vi "Main.vi"() -> ()   [LabVIEW 2017]
doc: "This Continuous Measurement sample project is based on the Queued Message Handler template.\n\nThe Event Handling Loop generates messages based on user interface actions.\n\nThe Message Handling Loop processes messages generated by the Event Handling Loop, or by other messages. There are also Acquisition and Logging message handling loop subVIs, and a chart updating loop."
uses:
  Settings/Settings.ctl
  Acquisition/Hardware Configuration.ctl
  Acquisition/Signal Type.ctl
  Logging/Logging Configuration.ctl
  controls/UI Data.ctl
  controls/UI State.ctl
  3e1da0e8-c032-3fe2-cb30-6c3ce3a1e83f.vi
  support/Message Queue/Enqueue Message (Single).vi
  support/Message Queue/Enqueue Message (Array).vi
  <vilib>/Utility/error.llb/Error Cluster From Error Code.vi
  <vilib>/ErrorRing/Error Ring.xnode
  Acquisition/Acquisition.lvlib
  Logging/Logging.lvlib
  Settings/Settings.lvlib
  support/User Event - Stop/User Event - Stop.lvlib
  support/Message Queue/Message Queue.lvlib
  Settings/Settings Dialog.vi
panel:
  out "Zero run":bool
  in  "Zero run?":bool
  out "Max writing time to a file [min]":dbl
  out "Elapsed time":timestamp
  out "Test time zero run [s]":dbl
  out "Test time [s]":dbl
  in  "Start":bool
  in  "Stop":bool
  in  "Settings":bool
  out "Status":string
  in  "Exit":bool
  out "Log File Offsite Path":path
  out "Project code":string
  out "Offsite storage?":bool
  out "Log File Path":path
  out "Data":waveform(dbl)[](graph)
  # "Continuous Measurement Data Logger"
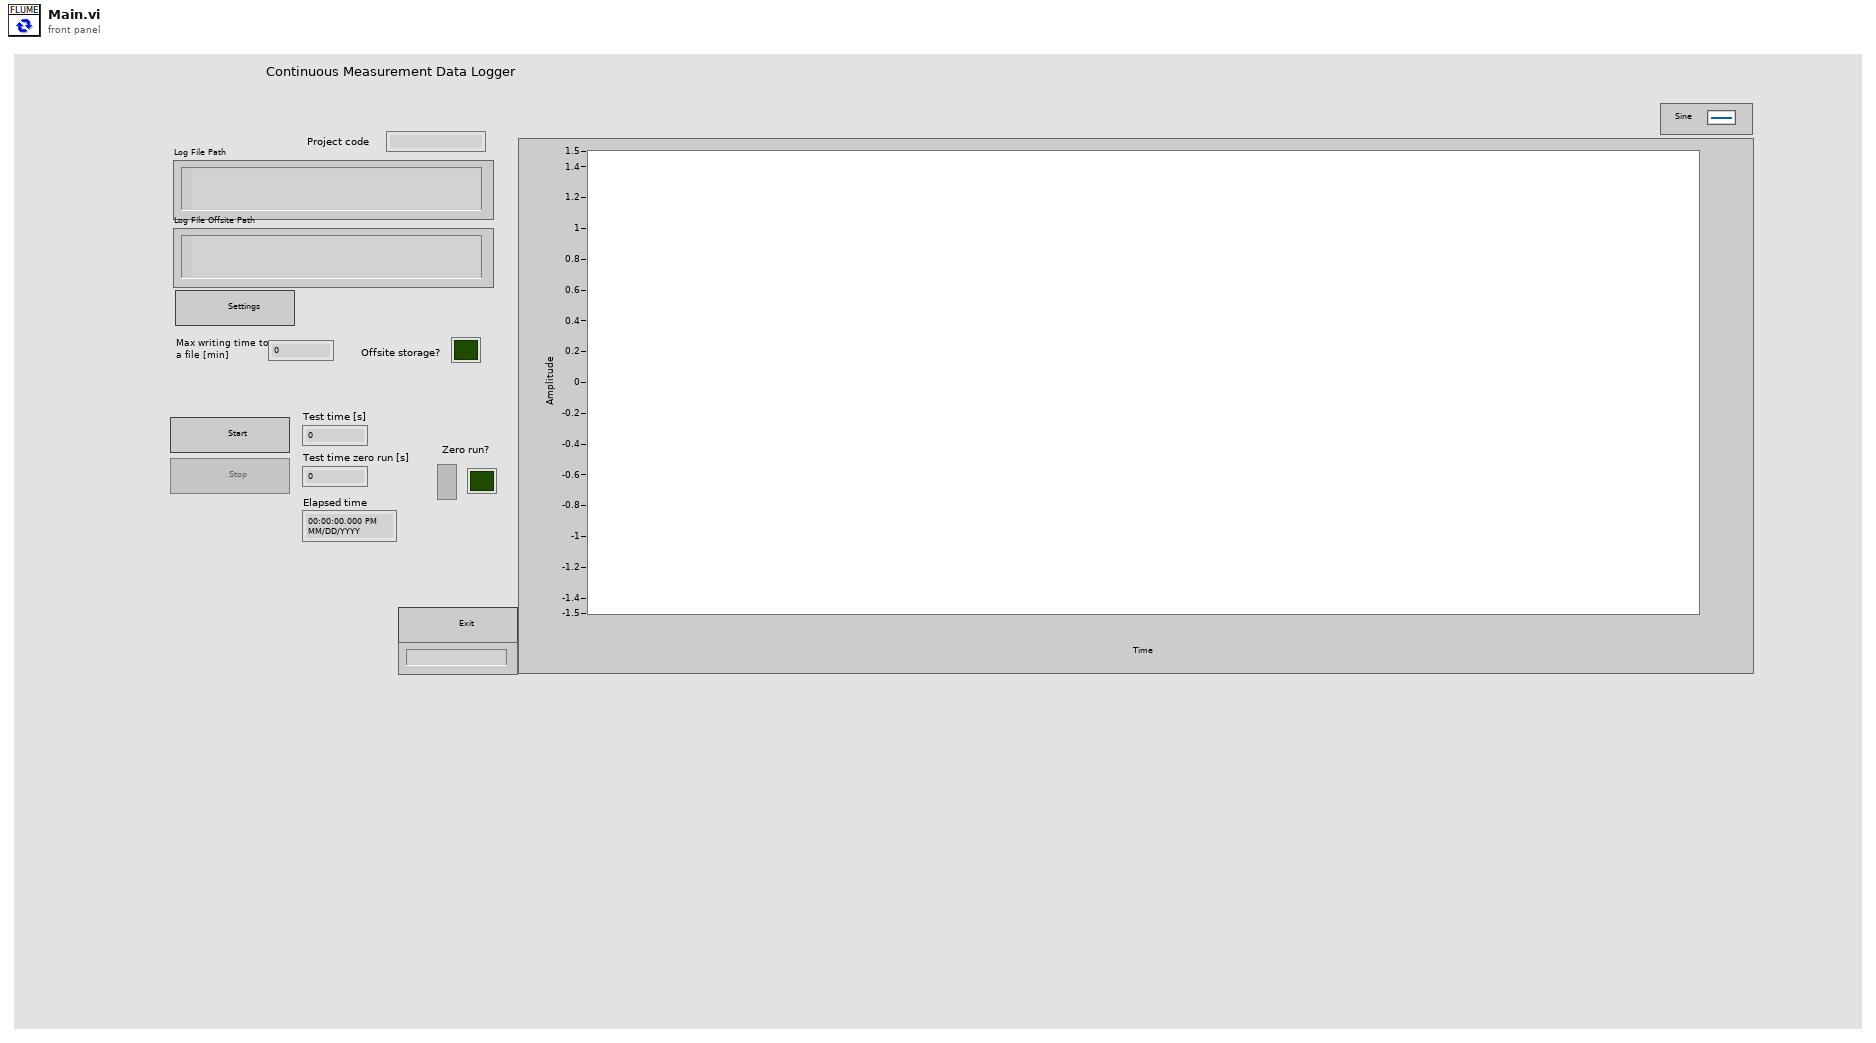
[diagram p1: front panel]
types:
  T1 = typedef "UI State.ctl" = enum16{"Idle", "Acquiring and Logging", "Waiting for Exit", "Waiting for Exit (Acq Stopped)", "Waiting for Exit (Log Stopped)", "Waiting for Stop", "Waiting for Stop (Acq Stopped)", "Waiting for Stop (Log Stopped)"}
  T2 = typedef "UI Data.ctl" = cluster{"Start Ref":refnum<vi>, "Stop Ref":refnum<vi>, "Settings Ref":refnum<vi>, "Exit Ref":refnum<vi>, "Status Ref":refnum<vi>, "Data Ref":refnum<vi>, "Zero run Ref":refnum<vi>}
  T3 = typedef "Settings.lvlib/Settings.ctl" = cluster{"Hardware Configuration":T4, "Logging Configuration":T6, "Cluster":cluster{"Elapsed Time":dbl, "Test time [s]":dbl, "Test time zero run[s] ":dbl, "Zero run?":bool}}
  T4 = typedef "Acquisition.lvlib/Hardware Configuration.ctl" = cluster{"HW Refnum <Replace Me>":string, "Signal Type <Replace Me>":T5}
  T5 = typedef "Acquisition.lvlib/Signal Type.ctl" = enum16{"Sine Wave", "Square with Noise"}
  T6 = typedef "Logging.lvlib/Logging Configuration.ctl" = cluster{"Log File Base Path":path, "TDMS File Reference":refnum<k34>, "Log File Offsite Path":path, "Offsite storage?":bool, "Project code":string, "Max writing time to a file [min]":dbl, "Bin File Reference":refnum<file>}
  T7 = typedef "Message Queue.lvlib/All Message Queues.ctl" = cluster{"UI":refnum<queue>, "Acquisition":refnum<queue>, "Logging":refnum<queue>, "Bin Logging":refnum<queue>}
  T8 = cluster{"Elapsed Time":dbl, "Test time [s]":dbl, "Test time zero run[s] ":dbl, "Zero run?":bool}
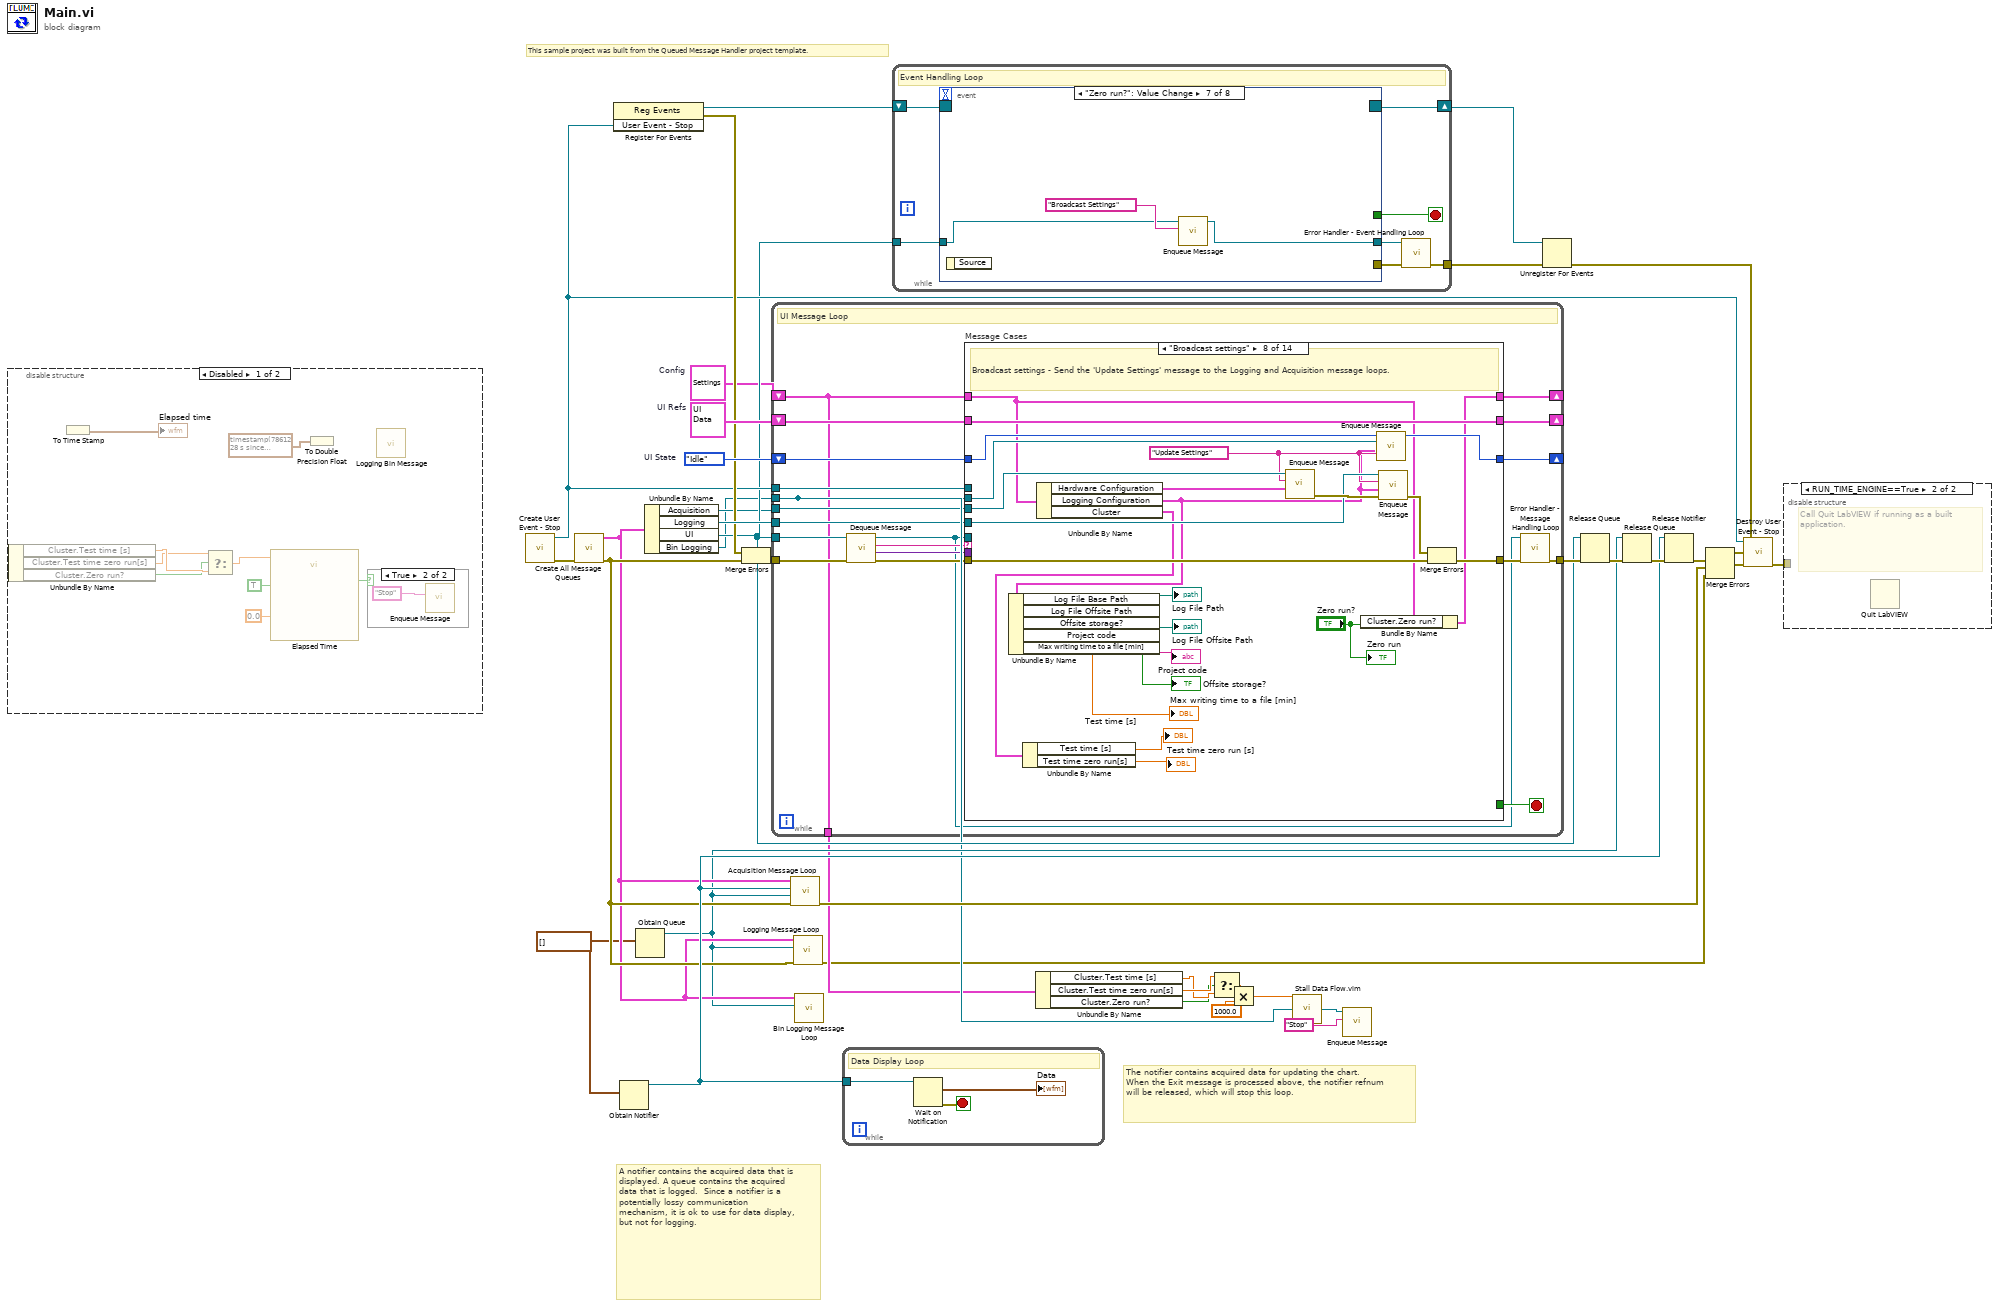
[diagram p0: block diagram]
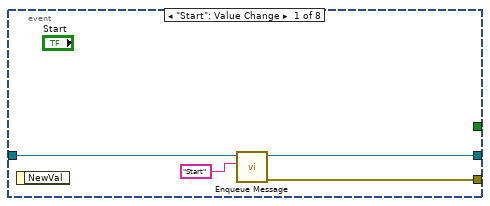
[diagram p5: hidden frame]
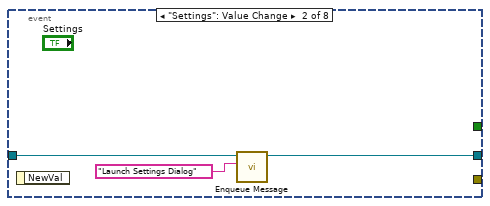
[diagram p6: hidden frame]
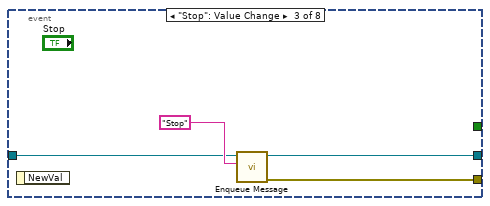
[diagram p7: hidden frame]
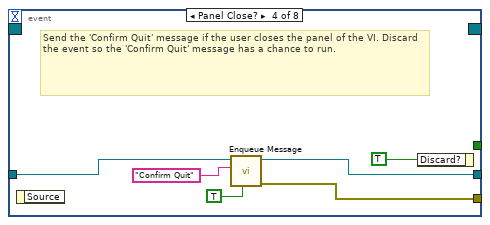
[diagram p8: hidden frame]
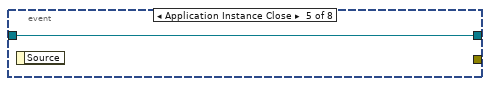
[diagram p9: hidden frame]
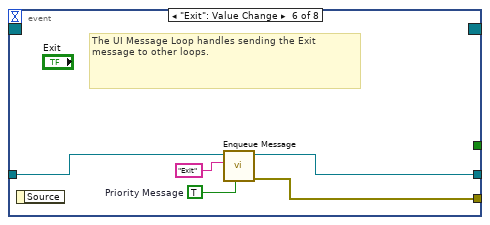
[diagram p10: hidden frame]
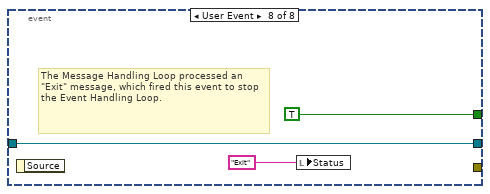
[diagram p11: hidden frame]
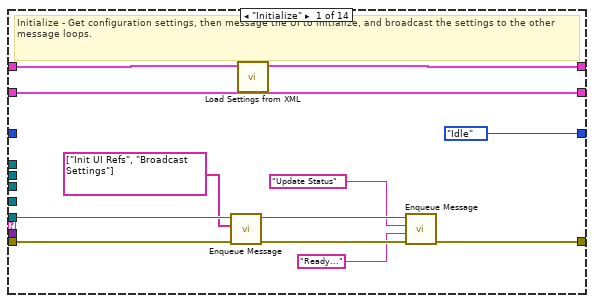
[diagram p12: hidden frame]
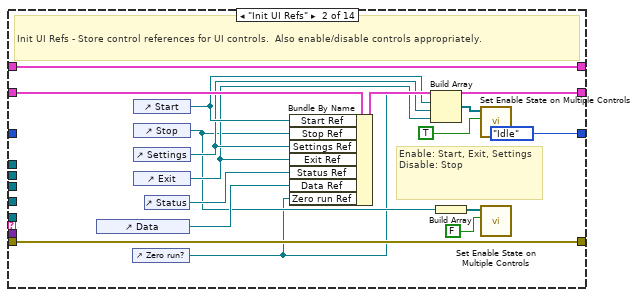
[diagram p13: hidden frame]
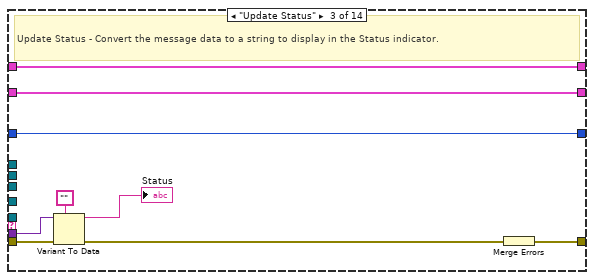
[diagram p14: hidden frame]
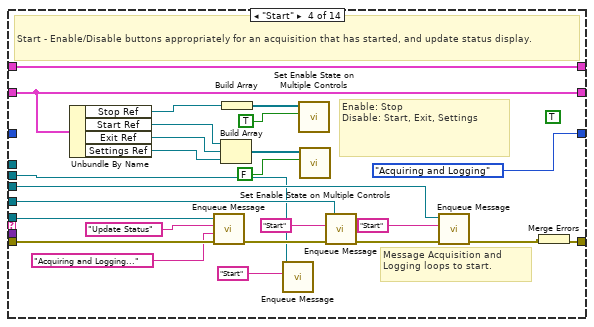
[diagram p15: hidden frame]
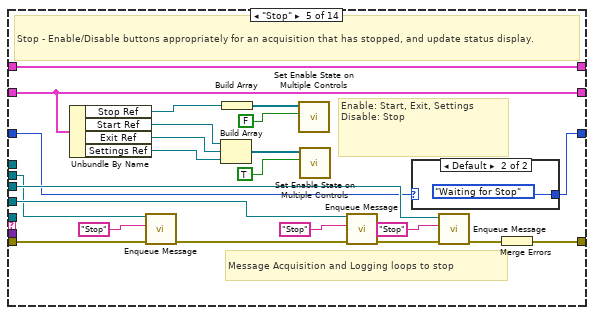
[diagram p16: hidden frame]
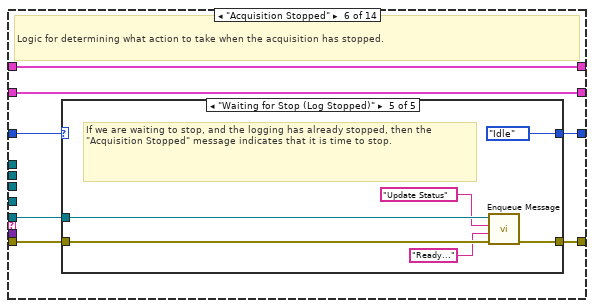
[diagram p18: hidden frame]
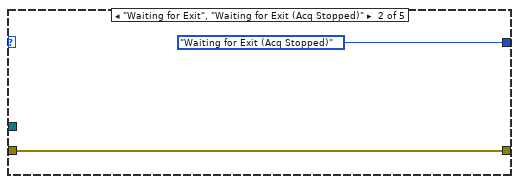
[diagram p20: hidden frame]
diagram:
  w31 = UI_State."Idle"  # UI State
  w14 = waveform(dbl)[] []
  w33 = T2 {"Start Ref"=refnum, "Stop Ref"=refnum, "Settings Ref"=refnum, "Exit Ref"=refnum, "Status Ref"=refnum, "Data Ref"=refnum, "Zero run Ref"=refnum}  # UI Refs
  w17 = T3 {"Hardware Configuration"={"HW Refnum <Replace Me>"="", "Signal Type <Replace Me>"=enum."Sine Wave"}, "Logging Configuration"={"Log File Base Path"=path "", "TDMS File Reference"=refnum, "Log File Offsite Path"=path "", "Offsite storage?"=FALSE, "Project code"="", "Max writing time to a file [min]"=0.0, "Bin File Reference"=refnum}, "Cluster"={"Elapsed Time"=0.0, "Test time [s]"=0.0, "Test time zero run[s] "=0.0, "Zero run?"=FALSE}}  # Config
  # "This sample project was built from the Queued Message Handler project template."
  # "A notifier contains the acquired data that is displayed. A queue contains the acquired data that is logged.  Since a notifier is a potentially lossy communication mechanism, it is ok to use for data display, but not for logging."
  # "The notifier contains acquired data for updating the chart. When the Exit message is processed above, the notifier refnum will be released, which will stop this loop."
  n1 = disable-structure shown="Disabled" {
    frame Disabled {
      n2 = Unbundle By Name() -> ("Cluster.Test time [s]"=w45:dbl, "Cluster.Test time zero run[s]"=w43:dbl, "Cluster.Zero run?"=w42:bool)  [unwired: 1 in]
      n3 = To Time Stamp() -> (0:→"Elapsed time":timestamp)  [unwired: 1 in]
      n4 = Select(t=w43, s=w42, f=w45) -> (s? t:f=w44:dbl)
      n5 = call "Elapsed Time"("Time Target (s)"=w44, "Auto Reset"=TRUE, "Set Start Time (s)"=0.0) -> ("Time has Elapsed"=w41:bool)  [unwired: 9 in, 7 out]
      n6 = To Double Precision Float(number=timestamp(7861228 s since 1904-01-01)) -> ()  [unwired: 1 out]
      n7 = case shown="True" w41 {
        frame False {
        }
        frame True {
          n8 = call-poly "Enqueue Message.vi"("Message"="Stop") -> ()  [unwired: 9 in, 2 out]
        }
      }
      n9 = call "Logging Bin Message.vi"() -> ()  [unwired: 11 in, 1 out]
    }
    frame Enabled {
    }
  }
  n10 = call "Create User Event - Stop.vi"() -> ("error out"=w35:errorcluster, "User Event - Stop"=w22:refnum<user-event>)  [unwired: 10 in]
  n11 = call "Create All Message Queues.vi"("error in (no error)"=w35) -> ("error out"=w16:errorcluster, "Message Queues out"=w15:T7)  [unwired: 9 in]
  n12 = register-events(w22) -> (reference out=w25:refnum<event-registration>, error out=w23:errorcluster)  [unwired: 2 in]
  n13 = Obtain Notifier(notification data type=w14) -> (notifier out=w18:refnum<notifier>)  [unwired: 3 in, 2 out]
  n14 = Obtain Queue(element data type=w14) -> (queue out=w13:refnum<queue>)  [unwired: 4 in, 2 out]
  n15 = Unbundle By Name(w15) -> ("Acquisition"=w20:refnum<queue>, "Logging"=w32:refnum<queue>, "UI"=w21:refnum<queue>, "Bin Logging"=w12:refnum<queue>)
  n16 = Merge Errors(w23, w16) -> (w24:errorcluster)
  n17 = while {
    tunnel: w21 -> [w53]
    tunnel: w22 -> [w66]
    shift-right: [w61] -> _
    shift-left: w17 -> [w49]
    shift-right: [w59] -> _
    shift-left: w33 -> [w60]
    tunnel: w20 -> [w58]
    tunnel: w32 -> [w52]
    shift-right: [w54] -> _
    shift-left: w31 -> [w55]
    tunnel: w24 -> [w65]
    tunnel: [w57] -> w38
    tunnel: w12 -> [w50]
    tunnel: [w50] -> w6
    tunnel: [w49] -> w4
    stop <- w67 stop-if-true
    # "UI Message Loop"
    n18 = call "Dequeue Message.vi"("error in (no error)"=w65, "Message Queue"=w53) -> ("error out"=w64:errorcluster, "Message Data"=w62:variant, "Message"=w63:string, "dup Message Queue"=w51:refnum<queue>)  [unwired: 6 in]
    n19 = case "Message Cases" shown="\"Broadcast settings\"" w63 {
      selector: w63 -> [_ _ _ _ _ _ _ _ _ _ _ _ _ w302]
      tunnel: w51 -> [w72 _ _ w108 _ w157 w182 _ w232 _ w254 _ _ _]
      tunnel: w64 -> [w71 w95 w103 w129 w150 w158 w183 w222 w234 w242 w253 w286 w300 _]
      tunnel: [w76 w95 w104 w110 w151 w155 w180 w226 w228 w245 w252 w293 w299 w301] -> w56
      tunnel: [_ _ _ _ _ _ _ _ _ _ _ TRUE _ _] -> w67
      tunnel: w62 -> [_ _ w102 _ _ _ _ _ _ w246 _ w284 _ _]
      tunnel: w66 -> [_ _ _ _ _ _ _ _ _ _ _ w294 _ _]
      tunnel: [w79 w82 w96 w106 w132 w154 w179 w204 w227 w241 w250 w282 w298 w305] -> w61
      tunnel: w49 -> [w68 w82 w96 w106 w132 w154 w179 w206 w235 w241 w250 w282 w298 w305]
      tunnel: w60 -> [w73 w94 w98 w126 w149 w160 w185 w221 w230 w249 w256 w292 w297 w304]
      tunnel: [w73 w91 w98 w126 w149 w160 w185 w221 w230 w249 w256 w292 w297 w304] -> w59
      tunnel: w58 -> [_ _ _ w109 w136 _ _ w220 _ _ _ w291 _ _]
      tunnel: w52 -> [_ _ _ w115 w139 _ _ w219 _ _ _ w290 _ _]
      tunnel: w55 -> [_ _ w97 _ w133 w159 w184 w218 w229 w244 w255 _ w296 w303]
      tunnel: [UI_State."Idle" ("UI State") UI_State."Idle" ("UI State") w97 UI_State."Acquiring and Logging" ("UI State") w134 w156 w181 w218 w229 w244 w251 UI_State."Idle" ("UI State") w296 w303] -> w54
      tunnel: w50 -> [_ _ _ w105 w130 _ _ w211 _ _ _ w281 _ _]
      frame "Initialize" {
        # "Initialize - Get configuration settings, then message the UI to initialize, and broadcast the settings to the other message loops."
        n20 = call-poly "Enqueue Message.vi"("error in (no error)"=w71, "Message Array"=string[] ["Init UI Refs", "Broadcast Settings"], "Message Queue"=w72) -> ("error out"=w78:errorcluster, "dup Message Queue"=w77:refnum<queue>)  [unwired: 7 in]
        n21 = call "Load Settings from XML.vi"("Settings in"=w68) -> ("Settings out"=w79:T3)  [unwired: 9 in, 1 out]
        n22 = call-poly "Enqueue Message.vi"("error in (no error)"=w78, "Message Data"="Ready..." ("Ready..."), "Message"="Update Status", "Message Queue"=w77) -> ("error out"=w76:errorcluster)  [unwired: 6 in, 1 out]
      }
      frame "Init UI Refs" {
        # "Enable: Start, Exit, Settings\nDisable: Stop"
        # "Init UI Refs - Store control references for UI controls.  Also enable/disable controls appropriately."
        n23 = control-ref of="Data"() -> (w92:refnum<vi>)
        n24 = control-ref of="Zero run?"() -> (w80:refnum<vi>)
        n25 = control-ref of="Start"() -> (w86:refnum<vi>)
        n26 = control-ref of="Stop"() -> (w81:refnum<vi>)
        n27 = control-ref of="Settings"() -> (w85:refnum<vi>)
        n28 = control-ref of="Exit"() -> (w84:refnum<vi>)
        n29 = control-ref of="Status"() -> (w93:refnum<vi>)
        n30 = Bundle By Name(cluster=w94, "Start Ref"=w86, "Stop Ref"=w81, "Settings Ref"=w85, "Exit Ref"=w84, "Status Ref"=w93, "Data Ref"=w92, "Zero run Ref"=w80) -> (w91:T2)
        n31 = Build Array(w80, w86, w85, w84) -> (w89:refnum<vi>[])
        n32 = Build Array(w81) -> (w88:refnum<vi>[])
        n33 = call "Set Enable State on Multiple Controls.vi"("Enable?"=TRUE, "Controls"=w89) -> ()  [unwired: 10 in]
        n34 = call "Set Enable State on Multiple Controls.vi"("Enable?"=FALSE, "Controls"=w88) -> ()  [unwired: 10 in]
      }
      frame "Update Status" {
        # "Update Status - Convert the message data to a string to display in the Status indicator."
        n35 = Variant To Data(error in=w103, type="", Variant=w102) -> (data=→"Status":string, error out=w100:errorcluster)
        n36 = Merge Errors(w100) -> (w104:errorcluster)
      }
      frame "Start" {
        (unwired) TRUE ("Reset")
        # "Message Acquisition and Logging loops to start."
        # "Enable: Stop\nDisable: Start, Exit, Settings"
        # "Start - Enable/Disable buttons appropriately for an acquisition that has started, and update status display."
        n37 = Unbundle By Name(w126) -> ("Stop Ref"=w121:refnum<vi>, "Start Ref"=w120:refnum<vi>, "Exit Ref"=w119:refnum<vi>, "Settings Ref"=w118:refnum<vi>)
        n38 = call-poly "Enqueue Message.vi"("error in (no error)"=w129, "Message Data"="Acquiring and Logging..." ("Acquiring and Logging..."), "Message"="Update Status", "Message Queue"=w108) -> ("error out"=w117:errorcluster)  [unwired: 6 in, 1 out]
        n39 = Build Array(w120, w119, w118) -> (w124:refnum<vi>[])
        n40 = Build Array(w121) -> (w123:refnum<vi>[])
        n41 = call-poly "Enqueue Message.vi"("Message"="Start", "Message Queue"=w105) -> ()  [unwired: 8 in, 2 out]
        n42 = call "Set Enable State on Multiple Controls.vi"("Enable?"=TRUE, "Controls"=w123) -> ()  [unwired: 10 in]
        n43 = call "Set Enable State on Multiple Controls.vi"("Enable?"=FALSE, "Controls"=w124) -> ()  [unwired: 10 in]
        n44 = call-poly "Enqueue Message.vi"("error in (no error)"=w117, "Message"="Start", "Message Queue"=w115) -> ("error out"=w112:errorcluster)  [unwired: 7 in, 1 out]
        n45 = call-poly "Enqueue Message.vi"("error in (no error)"=w112, "Message"="Start", "Message Queue"=w109) -> ("error out"=w111:errorcluster)  [unwired: 7 in, 1 out]
        n46 = Merge Errors(w111) -> (w110:errorcluster)
      }
      frame "Stop" {
        # "Message Acquisition and Logging loops to stop"
        # "Enable: Start, Exit, Settings\nDisable: Stop"
        # "Stop - Enable/Disable buttons appropriately for an acquisition that has stopped, and update status display."
        n47 = Unbundle By Name(w149) -> ("Stop Ref"=w144:refnum<vi>, "Start Ref"=w143:refnum<vi>, "Exit Ref"=w142:refnum<vi>, "Settings Ref"=w141:refnum<vi>)
        n48 = call-poly "Enqueue Message.vi"("Message"="Stop", "Message Queue"=w130) -> ()  [unwired: 8 in, 2 out]
        n49 = Build Array(w143, w142, w141) -> (w147:refnum<vi>[])
        n50 = Build Array(w144) -> (w146:refnum<vi>[])
        n51 = call "Set Enable State on Multiple Controls.vi"("Enable?"=FALSE, "Controls"=w146) -> ()  [unwired: 10 in]
        n52 = call "Set Enable State on Multiple Controls.vi"("Enable?"=TRUE, "Controls"=w147) -> ()  [unwired: 10 in]
        n53 = call-poly "Enqueue Message.vi"("error in (no error)"=w150, "Message"="Stop", "Message Queue"=w139) -> ("error out"=w138:errorcluster)  [unwired: 7 in, 1 out]
        n54 = case shown="Default" w133 {
          selector: w133 -> [w152 _]
          tunnel: [w152 UI_State."Waiting for Stop" ("UI State")] -> w134
          frame "Waiting for Exit" {
          }
          frame Default {
          }
        }
        n55 = call-poly "Enqueue Message.vi"("error in (no error)"=w138, "Message"="Stop", "Message Queue"=w136) -> ("error out"=w137:errorcluster)  [unwired: 7 in, 1 out]
        n56 = Merge Errors(w137) -> (w151:errorcluster)
      }
      frame "Acquisition Stopped" {
        # "Logic for determining what action to take when the acquisition has stopped."
        n57 = case shown="\"Waiting for Stop (Log Stopped)\"" w159 {
          selector: w159 -> [w162 _ _ _ _]
          tunnel: w158 -> [w161 w164 w166 w172 w178]
          tunnel: w157 -> [_ _ _ w170 w175]
          tunnel: [w162 UI_State."Waiting for Exit (Acq Stopped)" ("UI State") UI_State."Waiting for Stop (Acq Stopped)" ("UI State") UI_State."Idle" ("UI State") UI_State."Idle" ("UI State")] -> w156
          tunnel: [w161 w164 w166 w171 w176] -> w155
          frame Default {
          }
          frame "Waiting for Exit", "Waiting for Exit (Acq Stopped)" {
          }
          frame "Waiting for Stop", "Waiting for Stop (Acq Stopped)" {
          }
          frame "Waiting for Exit (Log Stopped)" {
            # "If we are waiting to exit, and the logging has already stopped, then the \"Acquisition Stopped\" message indicates that it is time to exit."
            n58 = call-poly "Enqueue Message.vi"("Priority Message? (F)"=TRUE, "error in (no error)"=w172, "Message"="Exit", "Message Queue"=w170) -> ("error out"=w171:errorcluster)  [unwired: 6 in, 1 out]
          }
          frame "Waiting for Stop (Log Stopped)" {
            # "If we are waiting to stop, and the logging has already stopped, then the \"Acquisition Stopped\" message indicates that it is time to stop."
            n59 = call-poly "Enqueue Message.vi"("error in (no error)"=w178, "Message Data"="Ready..." ("Ready..."), "Message"="Update Status", "Message Queue"=w175) -> ("error out"=w176:errorcluster)  [unwired: 6 in, 1 out]
          }
        }
      }
      frame "Logging Stopped" {
        # "Logic for determining what action to take when the logging has stopped."
        n60 = case shown="\"Waiting for Exit\", \"Waiting for Exit (Log Stopped)\"" w184 {
          selector: w184 -> [w187 _ _ _ _]
          tunnel: w183 -> [w186 w189 w191 w197 w200]
          tunnel: w182 -> [_ _ _ w195 w199]
          tunnel: [w187 UI_State."Waiting for Exit (Log Stopped)" ("UI State") UI_State."Waiting for Stop (Log Stopped)" ("UI State") UI_State."Idle" ("UI State") UI_State."Idle" ("UI State")] -> w181
          tunnel: [w186 w189 w191 w196 w198] -> w180
          frame Default {
          }
          frame "Waiting for Exit", "Waiting for Exit (Log Stopped)" {
          }
          frame "Waiting for Stop", "Waiting for Stop (Log Stopped)" {
          }
          frame "Waiting for Exit (Acq Stopped)" {
            # "If we are waiting to exit, and the acquisition has already stopped, then the \"Logging Stopped\" message indicates that it is time to exit."
            n61 = call-poly "Enqueue Message.vi"("Priority Message? (F)"=TRUE, "error in (no error)"=w197, "Message"="Exit", "Message Queue"=w195) -> ("error out"=w196:errorcluster)  [unwired: 6 in, 1 out]
          }
          frame "Waiting for Stop (Acq Stopped)" {
            # "If we are waiting to stop, and the acquisition has already stopped, then the \"Logging Stopped\" message indicates that it is time to stop."
            n62 = call-poly "Enqueue Message.vi"("error in (no error)"=w200, "Message Data"="Ready..." ("Ready..."), "Message"="Update Status", "Message Queue"=w199) -> ("error out"=w198:errorcluster)  [unwired: 6 in, 1 out]
          }
        }
      }
      frame "Broadcast settings" {
        w210 = "Update Settings" ("Message")
        # "Broadcast settings - Send the 'Update Settings' message to the Logging and Acquisition message loops."
        n63 = Unbundle By Name(w206) -> ("Hardware Configuration"=w224:T4, "Logging Configuration"=w209:T6, "Cluster"=w208:T8)
        n64 = Unbundle By Name(w209) -> ("Log File Base Path"=→"Log File Path":path, "Log File Offsite Path"=→"Log File Offsite Path":path, "Offsite storage?"=→"Offsite storage?":bool, "Project code"=→"Project code":string, "Max writing time to a file [min]"=→"Max writing time to a file [min]":dbl)
        n65 = Unbundle By Name(w208) -> ("Test time [s]"=→"Test time [s]":dbl, "Test time zero run[s]"=→"Test time zero run [s]":dbl)
        n66 = call-poly "Enqueue Message.vi"("Message Data"=w224, "Message"=w210, "Message Queue"=w220) -> ("error out"=w225:errorcluster)  [unwired: 7 in, 1 out]
        n67 = Bundle By Name(cluster=w206, "Cluster.Zero run?"="Zero run?") -> (w204:T3)
        n68 = call-poly "Enqueue Message.vi"("Message Data"=w209, "Message"=w210, "Message Queue"=w211) -> ()  [unwired: 7 in, 2 out]
        n69 = call-poly "Enqueue Message.vi"("error in (no error)"=w225, "Message Data"=w209, "Message"=w210, "Message Queue"=w219) -> ("error out"=w223:errorcluster)  [unwired: 6 in, 1 out]
        n70 = Merge Errors(w223, w222) -> (w226:errorcluster)
        "Zero run" <- "Zero run?"
      }
      frame "Launch Settings Dialog" {
        # "Launch Settings Dialog - Launch the Settings Dialog when the user clicks the 'Settings' button."
        n71 = call-by-ref "?"("error in (no error)"=w234, "Settings in"=w235) -> ("error out"=w231:errorcluster, "Cancelled?"=w233:bool, "Settings out"=w227:T3)  [unwired: 8 in, 3 out]
        n72 = case shown="False" w233 {
          tunnel: w232 -> [w239 _]
          tunnel: w231 -> [w238 w240]
          tunnel: [w237 w240] -> w228
          frame False {
            n73 = call-poly "Enqueue Message.vi"("error in (no error)"=w238, "Message"="Broadcast Settings", "Message Queue"=w239) -> ("error out"=w237:errorcluster)  [unwired: 7 in, 1 out]
          }
          frame True {
          }
        }
      }
      frame "Error" {
        # "Error - Display an error dialog. This message is sent by the \"Error Handler\" VIs at the end of other loops in this application."
        n74 = Variant To Data(error in=w242, type=errorcluster {"status"=FALSE, "code"=0, "source"=""} ("error constant"), Variant=w246) -> (data=w243:errorcluster, error out=w247:errorcluster)
        n75 = call <vilib>:"Simple Error Handler.vi"("error in (no error)"=w243) -> ()  [unwired: 4 in, 5 out]
        n76 = Merge Errors(w247) -> (w245:errorcluster)
      }
      frame "Confirm Quit" {
        # "Confirm Quit - Message that can confirm whether or not the user wants to exit the application."
        n77 = case shown="\"Acquiring and Logging\"" w255 {
          tunnel: w254 -> [w262 w266]
          tunnel: w253 -> [w261 w265]
          tunnel: [w260 w264] -> w252
          tunnel: [UI_State."Idle" ("UI State") w263] -> w251
          frame Default {
            # "If 'Confirm Quit' comes in while the system is idle, there is no need for a confirmation message."
            n78 = call-poly "Enqueue Message.vi"("Priority Message? (F)"=TRUE, "error in (no error)"=w261, "Message"="Exit", "Message Queue"=w262) -> ("error out"=w260:errorcluster)  [unwired: 6 in, 1 out]
          }
          frame "Acquiring and Logging" {
            n79 = Two Button Dialog(message="Are you sure you want to quit while the acquisition is running?" ("Confirm Quit Message"), 1:"No" ("No"), 2:"Yes" ("Yes")) -> (T button?=w267:bool)
            n80 = case shown="True" w267 {
              tunnel: w266 -> [_ w276]
              tunnel: w265 -> [w272 w277]
              tunnel: [w272 w275] -> w264
              tunnel: [UI_State."Acquiring and Logging" ("UI State") UI_State."Waiting for Exit" ("UI State")] -> w263
              frame False {
                # "User did not want to quit."
              }
              frame True {
                n81 = call-poly "Enqueue Message.vi"("error in (no error)"=w277, "Message"="Stop", "Message Queue"=w276) -> ("error out"=w275:errorcluster)  [unwired: 7 in, 1 out]
              }
            }
          }
        }
      }
      frame "Exit" {
        w287 = TRUE ("Priority Message? (F)")
        w280 = "Exit" ("Message")
        # "Popup an error dialog if 'Exit' was called as a result of an error."
        # "Stop the VI"
        # "Exit - Send Exit messages to the Acquisition and Logging loops, and fire the user event to stop the Event Handling Loop."
        n82 = Variant To Data(type=errorcluster {"status"=FALSE, "code"=0, "source"=""} ("error constant"), Variant=w284) -> (data=w283:errorcluster)  [unwired: 1 in, 1 out]
        n83 = call <vilib>:"Simple Error Handler.vi"("error in (no error)"=w283) -> ()  [unwired: 4 in, 5 out]
        n84 = call-poly "Enqueue Message.vi"("Priority Message? (F)"=w287, "error in (no error)"=w286, "Message"=w280, "Message Queue"=w291) -> ("error out"=w288:errorcluster)  [unwired: 6 in, 1 out]
        n85 = call-poly "Enqueue Message.vi"("Priority Message? (F)"=w287, "error in (no error)"=w288, "Message"=w280, "Message Queue"=w290) -> ("error out"=w279:errorcluster)  [unwired: 6 in, 1 out]
        n86 = call-poly "Enqueue Message.vi"("error in (no error)"=w279, "Message"=w280, "Message Queue"=w281) -> ("error out"=w278:errorcluster)  [unwired: 7 in, 1 out]
        n87 = call "Fire User Event - Stop.vi"("error in (no error)"=w278, "User Event - Stop"=w294) -> ("error out"=w293:errorcluster)  [unwired: 9 in]
      }
      frame "---Copy This Frame---" {
        (unwired) FALSE ("Time has Elapsed")
        # "Duplicate this frame when creating new messages.  Change this comment in the duplicated frame to describe this message."
        n88 = Merge Errors(w300) -> (w299:errorcluster)
      }
      frame Default {
        # "'Default' case only runs if there is a message that isn't defined in any of the other cases.  Output a programming error."
        n89 = xnode "Error Ring"("parameter 0"=w302) -> ("error out"=w301:errorcluster)
      }
    }
    n90 = call "Error Handler - Message Handling Loop.vi"("error in (no error)"=w56, "Message Queue"=w51) -> ("dup error in"=w57:errorcluster)  [unwired: 8 in, 1 out]
  }
  n91 = call "Acquisition Message Loop.vi"("error in (no error)"=w16, "Data Queue"=w13, "Data Notifier"=w18, "Message Queues"=w15) -> ("error out"=w36:errorcluster)  [unwired: 7 in]
  n92 = call "Logging Message Loop.vi"("error in (no error)"=w16, "Data Queue"=w13, "Message Queues"=w15) -> ("error out"=w3:errorcluster)  [unwired: 8 in]
  n93 = call "Bin Logging Message Loop.vi"("Data Queue"=w13, "Message Queues"=w15) -> ()  [unwired: 9 in, 1 out]
  n94 = while "Data Display Loop" {
    tunnel: w18 -> [w315]
    stop <- w314 stop-if-true
    # "Data Display Loop"
    n95 = Wait on Notification(notifier=w315) -> (notification=→"Data":waveform(dbl)[], error out=w314:errorcluster)  [unwired: 3 in, 2 out]
  }
  n96 = while {
    tunnel: w21 -> [w321]
    tunnel: [w318] -> w37
    shift-right: [w320] -> w34
    shift-left: w25 -> [w322]
    stop <- w319 stop-if-true
    # "Event Handling Loop"
    n97 = event shown="[6] \"Zero run?\": Value Change" {
      selector: w322 -> [_ _ _ _ _ _ _ _]
      dyn-events: [_ _ _ _ _ _ _ _] -> w320
      timeout: _ -> [_ _ _ _ _ _ _ _]
      tunnel: [_ _ _ _ _ _ _ TRUE ("Discard?")] -> w319
      tunnel: w321 -> [w326 w328 w332 w337 w340 w342 w347 w349]
      tunnel: [w324 _ w331 w335 _ w345 _ _] -> w317
      tunnel: [w323 w327 w330 w336 w340 w341 w346 w349] -> w316
      event "Start": Value Change {
        n98 = event-data() -> ()  [unwired: 1 in, 1 out]
        n99 = call-poly "Enqueue Message.vi"("Message"="Start", "Message Queue"=w326) -> ("error out"=w324:errorcluster, "dup Message Queue"=w323:refnum<queue>)  [unwired: 8 in]
      }
      event "Settings": Value Change {
        n100 = event-data() -> ()  [unwired: 1 in, 1 out]
        n101 = call-poly "Enqueue Message.vi"("Message"="Launch Settings Dialog", "Message Queue"=w328) -> ("dup Message Queue"=w327:refnum<queue>)  [unwired: 8 in, 1 out]
      }
      event "Stop": Value Change {
        n102 = event-data() -> ()  [unwired: 1 in, 1 out]
        n103 = call-poly "Enqueue Message.vi"("Message"="Stop", "Message Queue"=w332) -> ("error out"=w331:errorcluster, "dup Message Queue"=w330:refnum<queue>)  [unwired: 8 in]
      }
      event Panel Close? {
        # "Send the 'Confirm Quit' message if the user closes the panel of the VI. Discard the event so the 'Confirm Quit' message has a chance to run."
        n104 = event-data() -> ()  [unwired: 1 in, 1 out]
        n105 = call-poly "Enqueue Message.vi"("Priority Message? (F)"=TRUE, "Message"="Confirm Quit", "Message Queue"=w337) -> ("error out"=w335:errorcluster, "dup Message Queue"=w336:refnum<queue>)  [unwired: 7 in]
        n106 = event-data("Discard?"=TRUE) -> ()  [unwired: 1 in, 1 out]
      }
      event Application Instance Close {
        n107 = event-data() -> ()  [unwired: 1 in, 1 out]
      }
      event "Exit": Value Change {
        w343 = TRUE  # Priority Message
        # "The UI Message Loop handles sending the Exit message to other loops."
        n108 = event-data() -> ()  [unwired: 1 in, 1 out]
        n109 = call-poly "Enqueue Message.vi"("Priority Message? (F)"=w343, "Message"="Exit", "Message Queue"=w342) -> ("error out"=w345:errorcluster, "dup Message Queue"=w341:refnum<queue>)  [unwired: 7 in]
      }
      event "Zero run?": Value Change {
        n110 = event-data() -> ()  [unwired: 1 in, 1 out]
        n111 = call-poly "Enqueue Message.vi"("Message"="Broadcast Settings", "Message Queue"=w347) -> ("dup Message Queue"=w346:refnum<queue>)  [unwired: 8 in, 1 out]
      }
      event User Event {
        # "The Message Handling Loop processed an \"Exit\" message, which fired this event to stop the Event Handling Loop."
        n112 = event-data() -> ()  [unwired: 1 in, 1 out]
        n113 = local write "Status"("Exit" ("Exit String")) -> ()
      }
    }
    n114 = call "Error Handler - Event Handling Loop.vi"("error in (no error)"=w317, "Message Queue"=w316) -> ("dup error in"=w318:errorcluster)  [unwired: 8 in, 1 out]
  }
  n115 = Unbundle By Name(w4) -> ("Cluster.Test time [s]"=w2:dbl, "Cluster.Test time zero run[s]"=w8:dbl, "Cluster.Zero run?"=w1:bool)
  n116 = Select(t=w8, s=w1, f=w2) -> (s? t:f=w10:dbl)
  n117 = Multiply(x=w10, y=1000.0) -> (x*y=w11:dbl)
  n118 = call "Stall Data Flow.vim"("value in"=w6, "milliseconds to wait"=w11) -> ("value out"=w9:refnum<queue>)  [unwired: 1 out]
  n119 = call-poly "Enqueue Message.vi"("Message"="Stop", "Message Queue"=w9) -> ()  [unwired: 8 in, 2 out]
  n120 = Unregister For Events(event registration refnum=w34, error in=w37) -> (error out=w19:errorcluster)
  n121 = Release Queue(queue=w21, error in (no error)=w38) -> (error out=w28:errorcluster)  [unwired: 1 in, 2 out]
  n122 = Release Queue(queue=w13, error in (no error)=w28) -> (error out=w27:errorcluster)  [unwired: 1 in, 2 out]
  n123 = Release Notifier(notifier=w18, error in (no error)=w27) -> (error out=w26:errorcluster)  [unwired: 1 in, 2 out]
  n124 = Merge Errors(w19, w26, w36, w3) -> (w30:errorcluster)
  n125 = call "Destroy User Event - Stop.vi"("error in (no error)"=w30, "User Event - Stop"=w22) -> ("error out"=w29:errorcluster)  [unwired: 9 in]
  n126 = disable-structure shown="RUN_TIME_ENGINE==True" {
    disable-tunnel: w29 -> [_ _]
    frame condition #0 (active) {
    }
    frame condition #1 {
      # "Call Quit LabVIEW if running as a built application."
      n127 = Quit LabVIEW() -> ()  [unwired: 1 in]
    }
  }
